vi "获取宽和高.vi"(8 "错误输入（无错误）":errorcluster, 11 "引用":refnum<vi>) -> (0 "错误输出":errorcluster, 1 "高":i16, 2 "宽":i16, 3 "引用输出":refnum<vi>)   [LabVIEW 8.6, in "窗口操作.lvlib"]
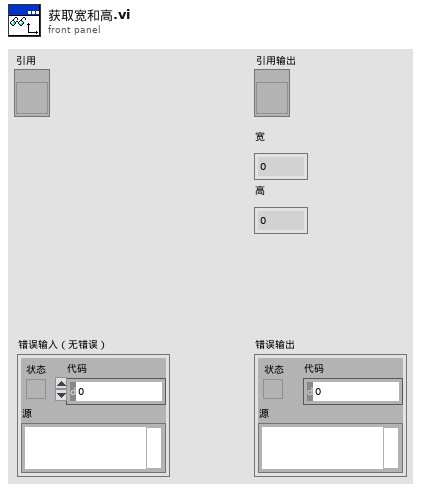
[diagram p1: front panel]
types:
  T1 = typedef "LVRectTypeDef.ctl" = cluster{"Left":i16, "Top":i16, "Right":i16, "Bottom":i16}
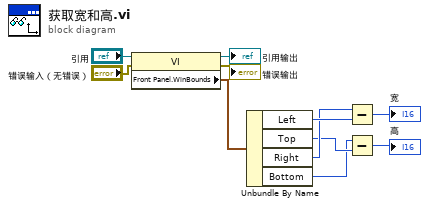
[diagram p0: block diagram]
diagram:
  n1 = property class="VI"(reference="引用", error in="错误输入（无错误）") -> (reference out=→"引用输出":refnum<vi>, error out=→"错误输出":errorcluster, "Front Panel.WinBounds"=w7:T1)
  n2 = Unbundle By Name(w7) -> ("Left"=w6:i16, "Top"=w4:i16, "Right"=w5:i16, "Bottom"=w3:i16)
  n3 = Subtract(x=w5, y=w6) -> (x-y=→"宽":i16)
  n4 = Subtract(x=w3, y=w4) -> (x-y=→"高":i16)
